vi "Main.vi"() -> ()   [LabVIEW 2015]
uses:
  Get File Information.lvlibp/control_Hierarchy.ctl
  Get File Information.lvlibp
  System.lvlibp
panel:
  in  "Hierarchy":T1 items=["root", "1", "2", "3"]
  in  "Check":bool
  in  "Listbox":i32(listbox)
  out "Table":string[][](table)
  in  "Path":path
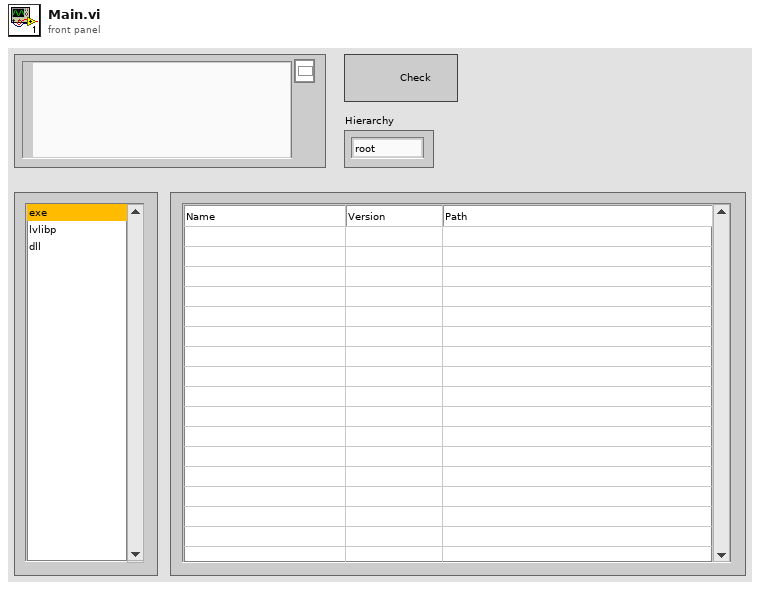
[diagram p1: front panel]
types:
  T1 = typedef "Get File Information.lvlibp/control_Hierarchy.ctl" = u16
  T2 = typedef "System.lvlibp/Control_Queue Reference.ctl" = refnum<queue>
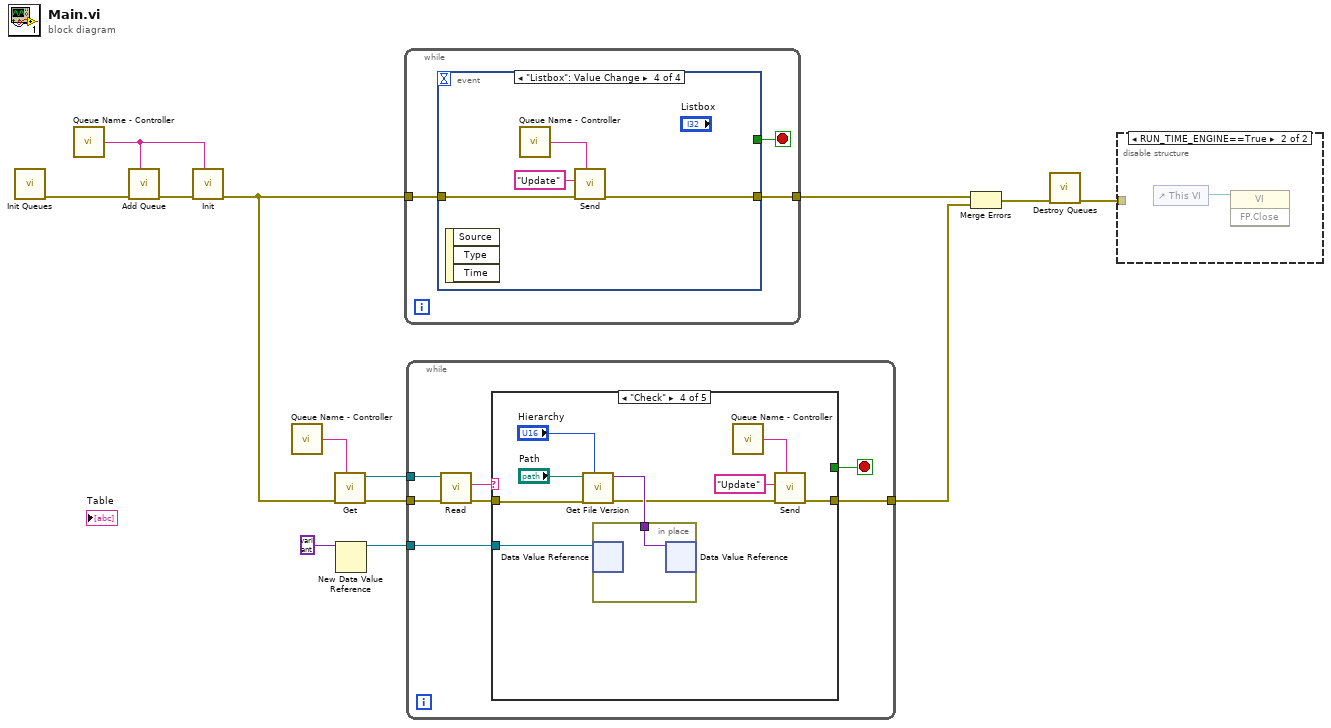
[diagram p0: block diagram]
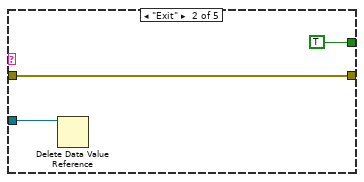
[diagram p4: hidden frame]
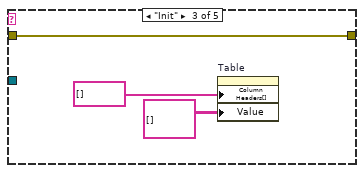
[diagram p5: hidden frame]
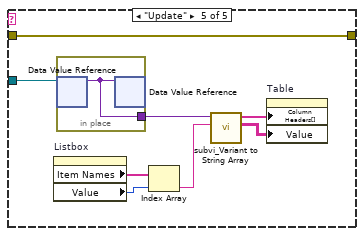
[diagram p6: hidden frame]
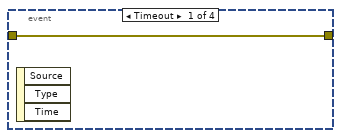
[diagram p7: hidden frame]
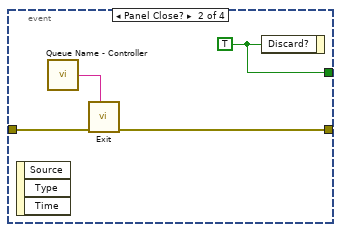
[diagram p8: hidden frame]
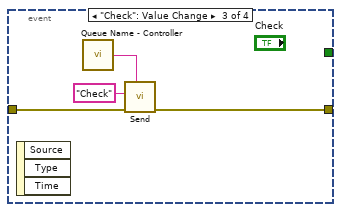
[diagram p9: hidden frame]
diagram:
  n1 = call "Init Queues.vi"() -> ("error out"=w13:errorcluster)  [unwired: 11 in]
  n2 = call "Queue Name - Controller.vi"() -> ("Queue Name"=w1:string)
  n3 = call "Add Queue.vi"("Process Name"=w1, "error in (no error)"=w13) -> ("error out"=w3:errorcluster)  [unwired: 9 in]
  n4 = call "Init.vi"("Process Name"=w1, "error in (no error)"=w3) -> ("error out"=w2:errorcluster)  [unwired: 9 in]
  n5 = call "Queue Name - Controller.vi"() -> ("Queue Name"=w12:string)
  n6 = call "Get.vi"("Process Name"=w12, "error in (no error)"=w2) -> ("error out"=w10:errorcluster, "queue out"=w11:T2)  [unwired: 8 in]
  n7 = New Data Value Reference(data value=variant) -> (data value reference=w5:refnum<data-value>)  [unwired: 1 in, 1 out]
  n8 = while {
    tunnel: w2 -> [w16]
    tunnel: [w14] -> w9
    stop <- w15 stop-if-true
    n9 = event shown="[3] \"Listbox\": Value Change" {
      selector: _ -> [_ _ _ _]
      dyn-events: _ -> [_ _ _ _]
      timeout: _ -> [_ _ _ _]
      tunnel: w16 -> [w17 w20 w25 w29]
      tunnel: [_ w21 _ _] -> w15
      tunnel: [w17 w18 w22 w28] -> w14
      event Timeout {
        n10 = event-data() -> ()  [unwired: 1 in, 3 out]
      }
      event Panel Close? {
        w21 = TRUE
        n11 = event-data() -> ()  [unwired: 1 in, 3 out]
        n12 = call "Queue Name - Controller.vi"() -> ("Queue Name"=w19:string)
        n13 = call "Exit.vi"("Process Name"=w19, "error in (no error)"=w20) -> ("error out"=w18:errorcluster)  [unwired: 9 in]
        n14 = event-data("Discard?"=w21) -> ()  [unwired: 1 in, 1 out]
      }
      event "Check": Value Change {
        n15 = event-data() -> ()  [unwired: 1 in, 3 out]
        n16 = call "Queue Name - Controller.vi"() -> ("Queue Name"=w24:string)
        n17 = call "Send.vi"("Process Name"=w24, "error in (no error)"=w25, "Message"="Check") -> ("error out"=w22:errorcluster)  [unwired: 8 in]
      }
      event "Listbox": Value Change {
        n18 = event-data() -> ()  [unwired: 1 in, 3 out]
        n19 = call "Queue Name - Controller.vi"() -> ("Queue Name"=w27:string)
        n20 = call "Send.vi"("Process Name"=w27, "error in (no error)"=w29, "Message"="Update") -> ("error out"=w28:errorcluster)  [unwired: 8 in]
      }
    }
  }
  n21 = while {
    tunnel: w11 -> [w36]
    tunnel: w10 -> [w35]
    tunnel: [w32] -> w8
    tunnel: w5 -> [w30]
    stop <- w31 stop-if-true
    n22 = call "Read.vi"("error in (no error)"=w35, "queue out"=w36) -> ("error out"=w33:errorcluster, "Message"=w34:string)  [unwired: 5 in, 3 out]
    n23 = case shown="\"Check\"" w34 {
      tunnel: w33 -> [w37 w39 w43 w51 w61]
      tunnel: [w37 w39 w43 w47 w61] -> w32
      tunnel: [_ TRUE _ _ _] -> w31
      tunnel: w30 -> [_ w38 _ w50 w60]
      frame Default {
      }
      frame "Exit" {
        n24 = Delete Data Value Reference(data value reference=w38) -> ()  [unwired: 1 in, 2 out]
      }
      frame "Init" {
        n25 = property on="Table" class="Tbl (strict)"("Column Headers[]"=string[] [] ("Column Header Strings[]"), "Value"=string[][] [] ("Table")) -> ()  [unwired: 2 in, 2 out]
      }
      frame "Check" {
        n26 = call "Get File Version.vi"("Hierarchy"="Hierarchy", "error in (no error)"=w51, "Folder Path"="Path") -> ("error out"=w48:errorcluster, "File Information"=w49:variant)  [unwired: 7 in]
        n27 = in-place {
          in-place-border: w49 -> [w53]
          n28 = in-place-dvr #1(w50) -> ()  [unwired: 2 out]
          n29 = in-place-dvr #1(w53) -> ()  [unwired: 2 out]
        }
        n30 = call "Queue Name - Controller.vi"() -> ("Queue Name"=w46:string)
        n31 = call "Send.vi"("Process Name"=w46, "error in (no error)"=w48, "Message"="Update") -> ("error out"=w47:errorcluster)  [unwired: 8 in]
      }
      frame "Update" {
        n32 = property on="Listbox" class="LstBox (strict)"() -> ("Item Names"=w56:string[], "Value"=w54:i32)  [unwired: 2 in, 2 out]
        n33 = in-place {
          in-place-border: [w62] -> w59
          n34 = in-place-dvr #2(w60) -> (w62:variant)  [unwired: 1 out]
          n35 = in-place-dvr #2(w62) -> ()  [unwired: 2 out]
        }
        n36 = Index Array(array=w56, index=w54) -> (element=w55:string)
        n37 = call "subvi_Variant to String Array.vi"("File Type"=w55, "Variant"=w59) -> ("File Information"=w57:string[][], "Header"=w58:string[])  [unwired: 8 in]
        n38 = property on="Table" class="Tbl (strict)"("Column Headers[]"=w58, "Value"=w57) -> ()  [unwired: 2 in, 2 out]
      }
    }
  }
  n39 = Merge Errors(w9, w8) -> (w7:errorcluster)
  n40 = call "Destroy Queues.vi"("error in (no error)"=w7) -> ("error out"=w4:errorcluster)  [unwired: 10 in]
  n41 = disable-structure shown="RUN_TIME_ENGINE==True" {
    disable-tunnel: w4 -> [_ _]
    frame condition #0 (active) {
    }
    frame condition #1 {
      n42 = control-ref of="This VI"() -> (w63:refnum<vi>)
      n43 = invoke class="VI" method="FP.Close"(reference=w63) -> ()  [unwired: 2 in, 3 out]
    }
  }
